vi "ExCameraNadvdisp.vi"() -> ()   [LabVIEW 2010]
panel:
  in  "done flag":bool
  in  "Exposure":dbl=0.01 min=0.0 step=0.01 format="%.2f"
  out "error out":errorcluster
  in  "error in (no error)":errorcluster
  in  "SITKFULLDISPLAYLib.SITKFullDisplay":refnum<k7>(container)
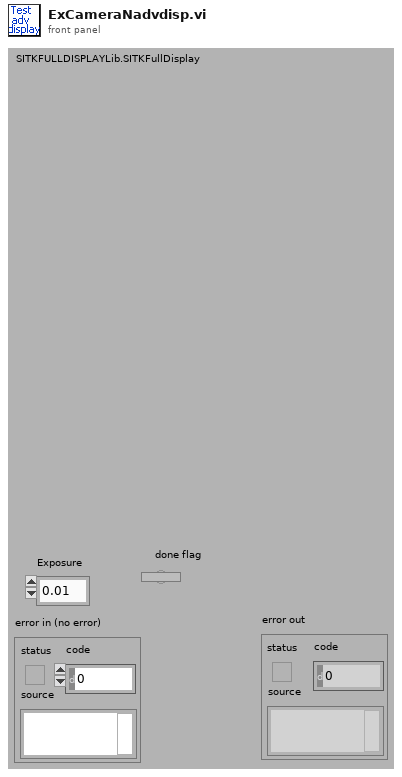
[diagram p1: front panel]
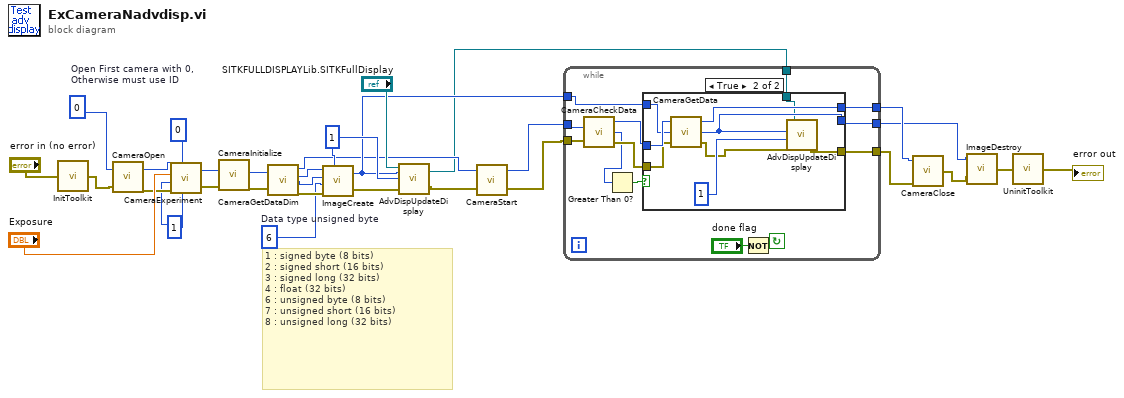
[diagram p0: block diagram]
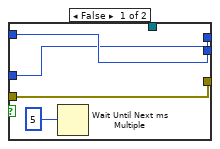
[diagram p2: hidden frame]
diagram:
  w14 = 6  # Data type unsigned byte
  w23 = 1
  w28 = 0  # Open First camera with 0, Otherwise must use ID
  w31 = 1
  # "1 : signed byte (8 bits)\n2 : signed short (16 bits)\n3 : signed long (32 bits)\n4 : float (32 bits)\n6 : unsigned byte (8 bits)\n7 : unsigned short (16 bits)\n8 : unsigned long (32 bits)"
  n1 = call <userlib>:"InitToolkit.vi"("error in"="error in (no error)") -> ("error out"=w27:errorcluster)
  n2 = call <userlib>:"CameraOpen.vi"("error in"=w27, "Camera Device ID"=w28) -> ("error out"=w24:errorcluster, "Camera Handle"=w25:u32)
  n3 = call <userlib>:"CameraExperiment.vi"("Number of Accumulations"=w23, "Acquire / Focus Flag"=0, "error in"=w24, "Number of Images"=w23, "Exposure (sec)"="Exposure", "Camera Handle"=w25) -> ("error out"=w21:errorcluster, "Camera Handle"=w20:u32)
  n4 = call <userlib>:"CameraInitialize.vi"("error in"=w21, "Camera Handle"=w20) -> ("error out"=w19:errorcluster, "Camera Handle"=w18:u32)
  n5 = call <userlib>:"CameraGetDataDim.vi"("Camera Handle"=w18, "error in"=w19) -> ("Camera Handle"=w10:u32, "Xdim"=w16:u32, "Ydim"=w15:u32, "error out"=w17:errorcluster)
  n6 = call <userlib>:"ImageCreate.vi"("X dimension"=w16, "Y dimension"=w15, "Data Type"=w14, "error in"=w17, "Number Of Frames"=w31) -> ("Image Handle"=w13:u32, "error out"=w12:errorcluster)
  n7 = call <userlib>:"AdvDispUpdateDisplay.vi"("error in (no error)"=w12, "Frame Number To Display"=w31, "Image Handle"=w13, "SITKFULLDISPLAYLib.SITKFullDisplay"="SITKFULLDISPLAYLib.SITKFullDisplay") -> ("error out"=w11:errorcluster, "SITKFULLDISPLAYLib.SITKFullDisplay"=w1:refnum<k7>)
  n8 = call <userlib>:"CameraStart.vi"("error in"=w11, "Camera Handle"=w10) -> ("error out"=w8:errorcluster, "Camera Handle"=w9:u32)
  n9 = while {
    tunnel: w9 -> [w37]
    tunnel: w8 -> [w36]
    tunnel: [w40] -> w5
    tunnel: [w39] -> w3
    tunnel: [w44] -> w6
    tunnel: w13 -> [w43]
    tunnel: w1 -> [w32]
    stop <- w41 continue-if-true
    n10 = call <userlib>:"CameraCheckData.vi"("Camera Handle"=w37, "error in"=w36) -> ("Camera Handle"=w35:u32, "Number Of Frames Available"=w33:i32, "error out"=w38:errorcluster)
    n11 = Greater Than 0?(x=w33) -> (x > 0?=w34:bool)
    n12 = case shown="True" w34 {
      tunnel: w35 -> [w46 w57]
      tunnel: w38 -> [w48 w56]
      tunnel: [w46 w55] -> w44
      tunnel: w43 -> [w47 w54]
      tunnel: [w48 w50] -> w40
      tunnel: [w47 w53] -> w39
      tunnel: w32 -> [_ w49]
      frame False {
        n13 = Wait Until Next ms Multiple(millisecond multiple=5) -> ()  [unwired: 1 out]
      }
      frame True {
        n14 = call <userlib>:"CameraGetData.vi"("error in"=w56, "Data Handle"=w54, "Camera Handle"=w57) -> ("error out"=w51:errorcluster, "Data Handle"=w53:u32, "Camera Handle"=w55:u32)
        n15 = call <userlib>:"AdvDispUpdateDisplay.vi"("error in (no error)"=w51, "Frame Number To Display"=1, "Image Handle"=w53, "SITKFULLDISPLAYLib.SITKFullDisplay"=w49) -> ("error out"=w50:errorcluster)  [unwired: 1 out]
      }
    }
    n16 = Not(x="done flag") -> (.not. x?=w41:bool)
  }
  n17 = call <userlib>:"CameraClose.vi"("error in"=w5, "Camera Handle"=w6) -> ("error out"=w4:errorcluster)
  n18 = call <userlib>:"ImageDestroy.vi"("error in"=w4, "Data handle"=w3) -> ("error out"=w7:errorcluster)
  n19 = call <userlib>:"UninitToolkit.vi"("error in"=w7) -> ("error out"=→"error out":errorcluster)
